vi "PPFS_SIM_Gyro_Open.vi"(8 "IMU CAN ID":u8) -> (0 "error out":errorcluster, 3 "Gyro Ref":T1)   [LabVIEW 2023]
uses:
  PPFS_SIM_SIM_Globals.vi
  <vilib>/Rock Robotics/WPI/ThirdParty/Phoenix6/getters/GetPigeon2Yaw.vi
  <vilib>/Rock Robotics/WPI/ThirdParty/Phoenix6/DeviceReference.ctl
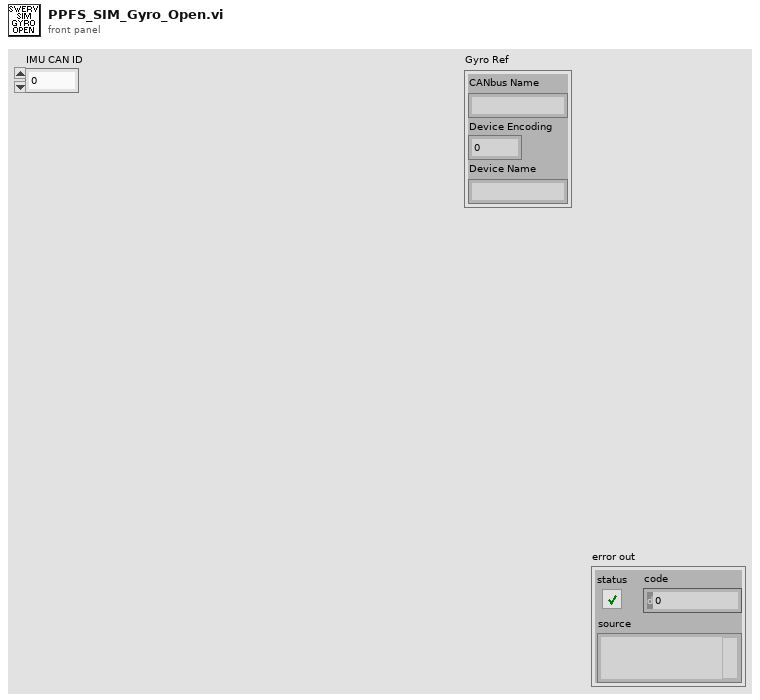
[diagram p1: front panel]
types:
  T1 = typedef "DeviceReference.ctl" = cluster{"CANbus Name":string, "Device Encoding":u32, "Device Name":string}
  T2 = cluster{"Value":dbl, "System Timestamp":dbl, "CANivore Timestamp":dbl, "ECU Timestamp":dbl}
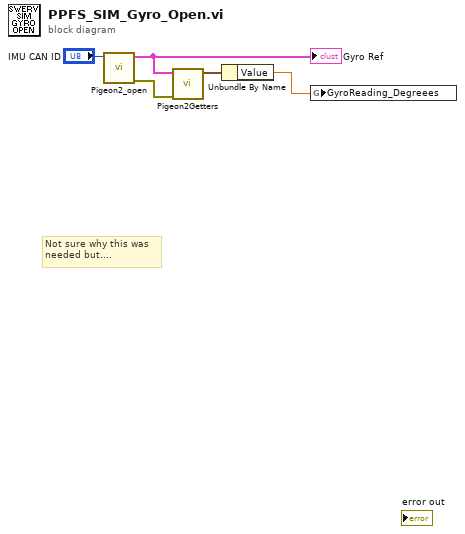
[diagram p0: block diagram]
diagram:
  # "Not sure why this was\nneeded but...."
  n1 = call <vilib>:"Pigeon2_open.vi"("Device ID"="IMU CAN ID") -> ("error out"=w4:errorcluster, "DeviceReference 2"=w3:T1)  [unwired: 9 in]
  "Gyro Ref" <- w3
  n2 = call-poly <vilib>:"Pigeon2Getters.vi"("error in"=w4, "DeviceReference"=w3) -> ("Output"=w2:T2)  [unwired: 8 in, 1 out]
  n3 = Unbundle By Name(w2) -> ("Value"=w1:dbl)
  n4 = global write "PPFS_SIM_SIM_Globals.vi" "GyroReading_Degreees"(w1) -> ()
